vi "Read Props.vi"(8 "error in (no error)":errorcluster, 11 "2WayValveEditorPanel in":refnum<class "2WayValveEditorPanel.lvclass">) -> (0 "error out":errorcluster, 2 "Props":T1, 3 "2WayValveEditorPanel out":refnum<class "2WayValveEditorPanel.lvclass">)   [LabVIEW 2020, in "VolatusGUIControls.lvlib" / "2WayValveEditorPanel.lvclass"]
uses:
  2WayValveEditorPanel.lvclass
  2WayValveEditorPanel.lvclass/2WayValveEditorPanel.ctl
  VolatusGUIControls.lvlib
  410f5dd6-b380-499c-a24f-4dc55d6ea509.vi
  JSON Props.ctl
  VolatusGUIEditorCore/Label Props.ctl
  VolatusGUIEditorCore/VolatusGUIEditorCore.lvlib
  VolatusGUIEditorCore/Position Props.ctl
  Props.ctl
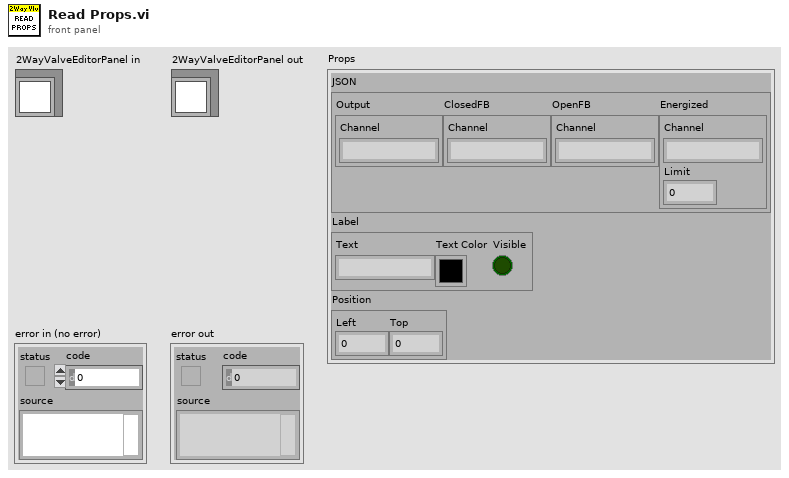
[diagram p1: front panel]
types:
  T1 = typedef "VolatusGUIControls.lvlib/2WayValveEditorPanel.lvclass/Props.ctl" = cluster{"JSON":T2, "Label":T3, "Position":T4}
  T2 = typedef "VolatusGUIControls.lvlib/2WayValveEditorPanel.lvclass/JSON Props.ctl" = cluster{"Output":cluster{"Channel":string}, "ClosedFB":cluster{"Channel":string}, "OpenFB":cluster{"Channel":string}, "Energized":cluster{"Channel":string, "Limit":dbl}}
  T3 = typedef "VolatusGUIEditorCore.lvlib/Label Props.ctl" = cluster{"Text":string, "Text Color":u32, "Visible":bool}
  T4 = typedef "VolatusGUIEditorCore.lvlib/Position Props.ctl" = cluster{"Left":i32, "Top":i32}
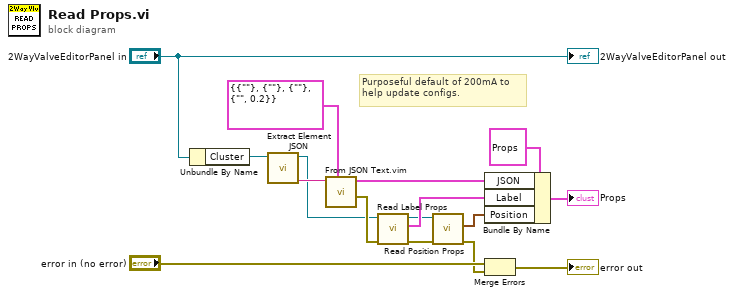
[diagram p0: block diagram]
diagram:
  # "Purposeful default of 200mA to help update configs."
  n1 = Unbundle By Name("2WayValveEditorPanel in") -> ("Cluster"=w13:refnum<vi>)
  n2 = call "Extract Element JSON.vi"("Ctl Refnum in"=w13) -> ("JSON"=w12:string, "Ctl Refnum"=w7:refnum<vi>)  [unwired: 7 in, 2 out]
  n3 = call "From JSON Text.vim"("Data Type and Default Value"=T2 {"Output"={"Channel"=""}, "ClosedFB"={"Channel"=""}, "OpenFB"={"Channel"=""}, "Energized"={"Channel"="", "Limit"=0.2}} ("JSON Props"), "JSON"=w12) -> ("error out"=w16:errorcluster, "Data out"=w8:T2)  [unwired: 8 in]
  n4 = call "Read Label Props.vi"("error in (no error)"=w16, "Ctl Refnum in"=w7) -> ("error out"=w4:errorcluster, "Label Props"=w6:T3, "Ctl Refnum"=w5:refnum<vi>)  [unwired: 7 in]
  n5 = call "Read Position Props.vi"("error in (no error)"=w4, "Ctl Refnum in"=w5) -> ("error out"=w1:errorcluster, "Position Props"=w3:T4)  [unwired: 7 in, 1 out]
  n6 = Bundle By Name(cluster=T1 {"JSON"={"Output"={"Channel"=""}, "ClosedFB"={"Channel"=""}, "OpenFB"={"Channel"=""}, "Energized"={"Channel"="", "Limit"=0.0}}, "Label"={"Text"="", "Text Color"=0, "Visible"=FALSE}, "Position"={"Left"=0, "Top"=0}} ("Props"), "JSON"=w8, "Label"=w6, "Position"=w3) -> (→"Props":T1)
  n7 = Merge Errors("error in (no error)", w1) -> (→"error out":errorcluster)
  "2WayValveEditorPanel out" <- "2WayValveEditorPanel in"
